vi "DAQ_Intial_Scope_AI3.vi"(8 "error in":errorcluster, 11 "physical channel":string="Dev7/ai3") -> (0 "error out":errorcluster, 3 "task out":refnum<k21>)   [LabVIEW 2015]
uses:
  <vilib>/DAQmx/configure/timing.llb/DAQmx Timing (Sample Clock).vi
  <vilib>/DAQmx/create/channels.llb/DAQmx Create Channel (AI-Voltage-Basic).vi
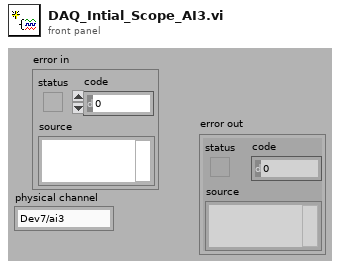
[diagram p1: front panel]
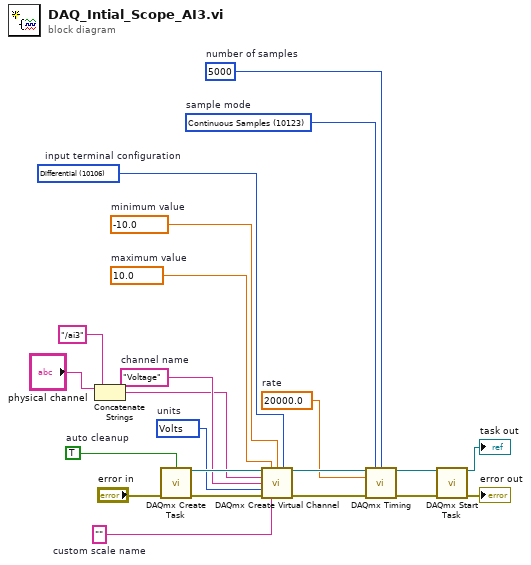
[diagram p0: block diagram]
diagram:
  w8 = 10123 items=["Finite Samples"=10178, "Continuous Samples"=10123, "Hardware Timed Single Point"=12522]  # sample mode
  w9 = 5000  # number of samples
  w10 = 20000.0  # rate
  w12 = 10106 items=["default"=-1, "RSE"=10083, "NRSE"=10078, "Differential"=10106, "Pseudodifferential"=12529]  # input terminal configuration
  w13 = 10348 items=["Volts"=10348, "From Custom Scale"=10065]  # units
  w14 = "Voltage"  # channel name
  w16 = ""  # custom scale name
  w17 = -10.0  # minimum value
  w18 = 10.0  # maximum value
  w20 = TRUE  # auto cleanup
  n1 = Concatenate Strings("physical channel", "/ai3" ("string")) -> (w1:string)
  n2 = call <vilib>:"DAQmx Create Task.vi"("auto cleanup"=w20, "error in"="error in") -> ("task out"=w19:refnum<k21>, "error out"=w21:errorcluster)  [unwired: 12 in]
  n3 = call-poly <vilib>:"DAQmx Create Virtual Channel.vi"("task in"=w19, "maximum value"=w18, "minimum value"=w17, "input terminal configuration"=w12, "physical channels"=w1, "name to assign"=w14, "units"=w13, "error in"=w21, "custom scale name"=w16) -> ("task out"=w11:refnum<k21>, "error out"=w15:errorcluster)  [unwired: 5 in]
  n4 = call-poly <vilib>:"DAQmx Timing.vi"("task/channels in"=w11, "sample mode"=w8, "samples per channel"=w9, "rate"=w10, "error in"=w15) -> ("task out"=w7:refnum<k21>, "error out"=w6:errorcluster)  [unwired: 9 in]
  n5 = call <vilib>:"DAQmx Start Task.vi"("task/channels in"=w7, "error in"=w6) -> ("task out"=→"task out":refnum<k21>, "error out"=→"error out":errorcluster)  [unwired: 12 in]
